vi "LVJSON Set.vi"(8 "error in (no error)":errorcluster, 10 "Root Element to Merge":T1, 11 "Root Element in":T1) -> (0 "error out":errorcluster, 2 "Exists?":bool, 3 "Root Element out":T1)   [LabVIEW 2019, in "labview_json.lvlib"]
uses:
  labview_json.lvlib
  Element.ctl
  Element Type.ctl
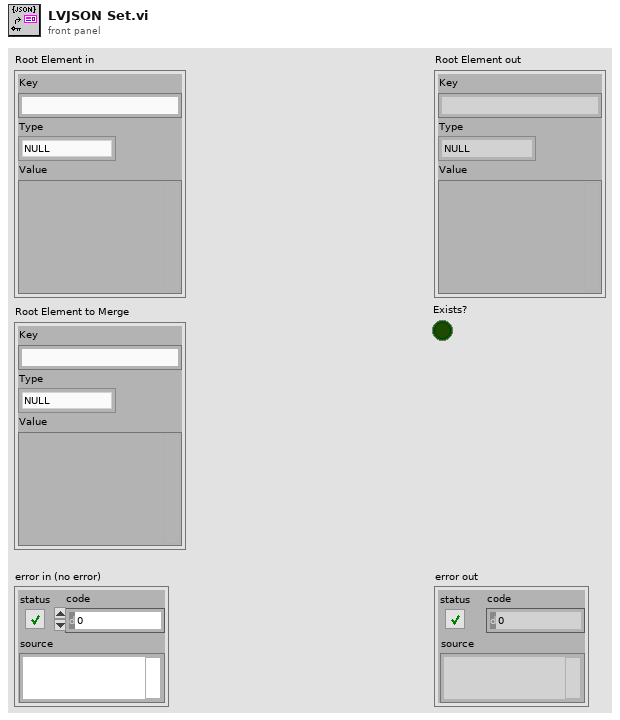
[diagram p1: front panel]
types:
  T1 = typedef "labview_json.lvlib/Element.ctl" = cluster{"Key":string, "Type":T2, "Value":variant}
  T2 = typedef "labview_json.lvlib/Element Type.ctl" = enum8{"NULL", "BOOL", "INT", "UINT", "FLOAT", "STRING", "ARRAY", "OBJECT", "SKIP"}
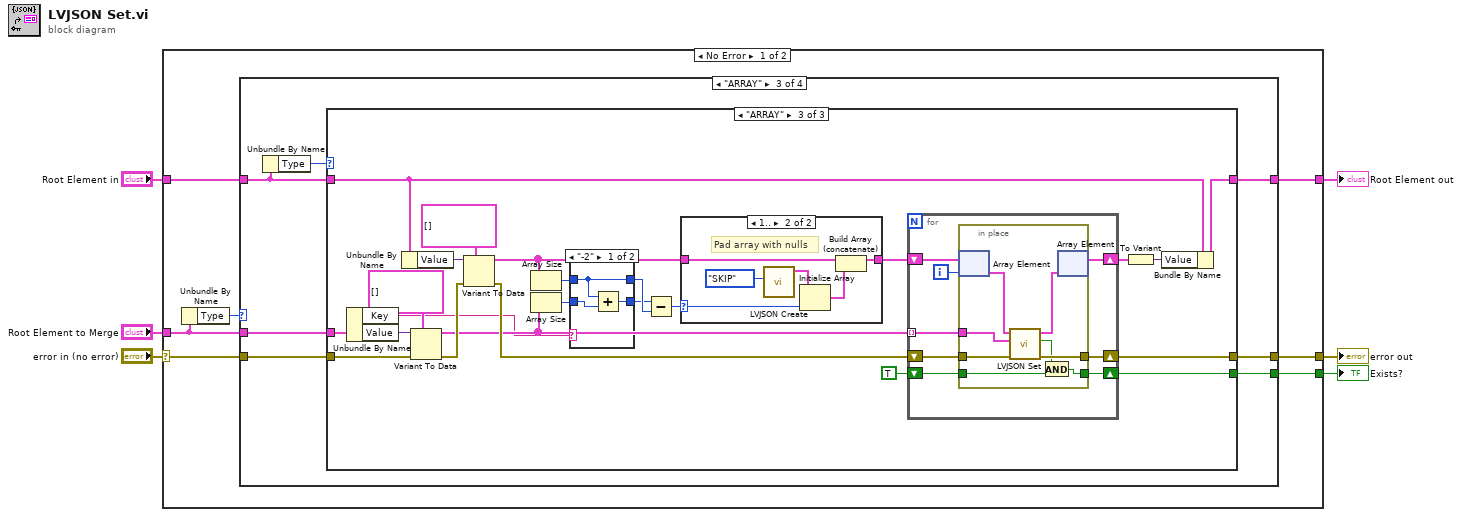
[diagram p0: block diagram]
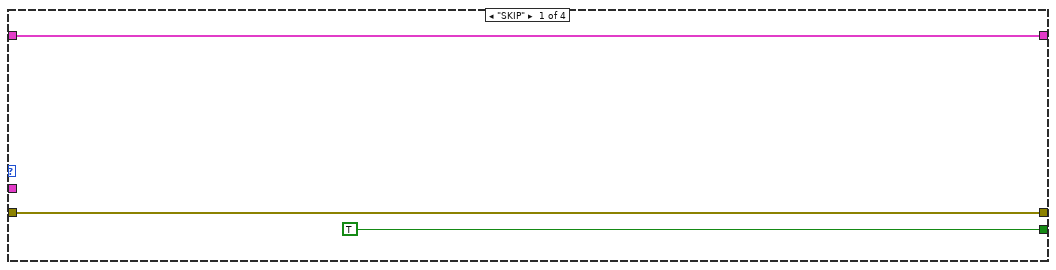
[diagram p2: hidden frame]
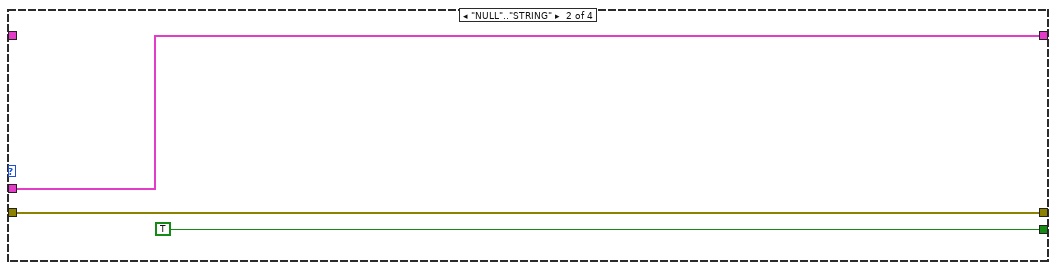
[diagram p3: hidden frame]
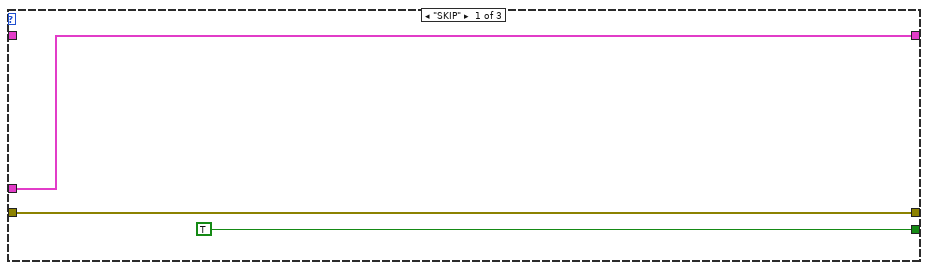
[diagram p4: hidden frame]
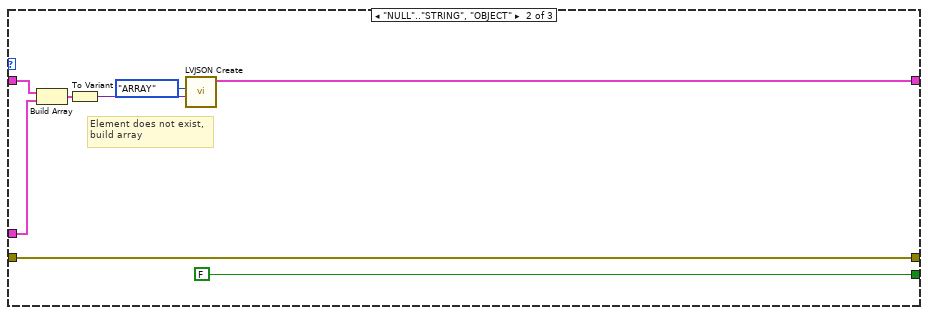
[diagram p5: hidden frame]
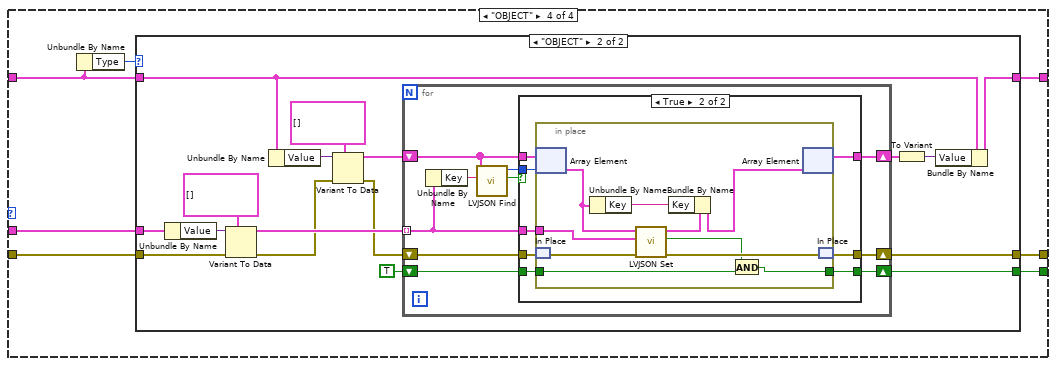
[diagram p8: hidden frame]
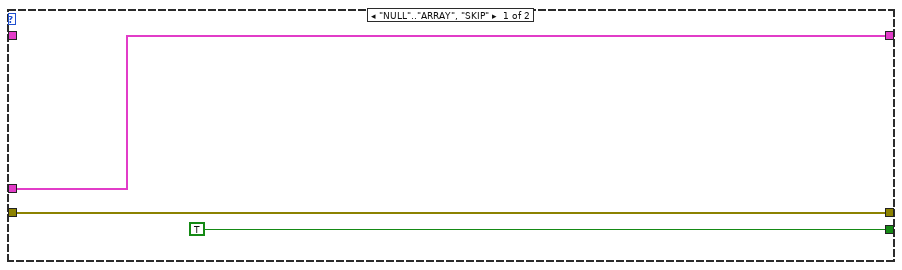
[diagram p9: hidden frame]
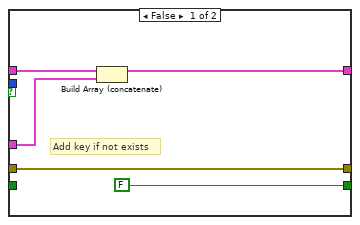
[diagram p10: hidden frame]
diagram:
  n1 = case shown="No Error" "error in (no error)" {
    selector: "error in (no error)" -> [w8 w151]
    tunnel: [w11 w151] -> w6
    tunnel: "Root Element in" -> [w13 w150]
    tunnel: "Root Element to Merge" -> [w7 _]
    tunnel: [w12 w150] -> w2
    tunnel: [w10 _] -> w1
    frame No Error {
      n2 = Unbundle By Name(w7) -> ("Type"=w9:T2)
      n3 = case shown="\"ARRAY\"" w9 {
        tunnel: w13 -> [w16 _ w22 w90]
        tunnel: [w16 w17 w25 w95] -> w12
        tunnel: w7 -> [_ w17 w20 w93]
        tunnel: w8 -> [w15 w19 w21 w91]
        tunnel: [w15 w19 w26 w96] -> w11
        tunnel: [TRUE ("Exists?") TRUE ("Exists?") w24 w94] -> w10
        frame "SKIP" {
        }
        frame "NULL".."STRING" {
        }
        frame "ARRAY" {
          n4 = Unbundle By Name(w22) -> ("Type"=w23:T2)
          n5 = case shown="\"ARRAY\"" w23 {
            tunnel: w22 -> [_ w37 w54]
            tunnel: w21 -> [w28 w36 w47]
            tunnel: [w28 w36 w61] -> w26
            tunnel: [w29 w35 w60] -> w25
            tunnel: [TRUE ("Exists?") FALSE ("Exists?") w59] -> w24
            tunnel: w20 -> [w29 w30 w46]
            frame "SKIP" {
            }
            frame "NULL".."STRING", "OBJECT" {
              # "Element does not exist,\nbuild array"
              n6 = Build Array(w37, w30) -> (w33:T1[])
              n7 = To Variant(anything=w33) -> (Variant=w32:variant)
              n8 = call "LVJSON Create.vi"("Variant (Void=Default Type)"=w32, "Type"=Element_Type."ARRAY") -> ("Element out"=w35:T1)  [unwired: 9 in]
            }
            frame "ARRAY" {
              n9 = Unbundle By Name(w46) -> ("Key"=w42:string, "Value"=w51:variant)
              n10 = Unbundle By Name(w54) -> ("Value"=w58:variant)
              n11 = Variant To Data(error in=w47, type=T1[] [], Variant=w51) -> (data=w48:T1[], error out=w49:errorcluster)
              n12 = Variant To Data(error in=w49, type=T1[] [], Variant=w58) -> (data=w53:T1[], error out=w52:errorcluster)
              n13 = Array Size(array=w53) -> (size(s)=w40:i32)
              n14 = Array Size(array=w48) -> (size(s)=w38:i32)
              n15 = case shown="\"-2\"" w42 {
                tunnel: [w63 w66] -> w41
                tunnel: w40 -> [w63 w66]
                tunnel: [w64 w65] -> w39
                tunnel: w38 -> [w62 w65]
                frame "-2" {
                  n16 = Add(x=w63, y=w62) -> (x+y=w64:i32)
                }
                frame Default {
                }
              }
              n17 = Subtract(x=w39, y=w41) -> (x-y=w44:i32)
              n18 = case shown="1.." w44 {
                selector: w44 -> [_ w68]
                tunnel: w53 -> [w67 w70]
                tunnel: [w67 w69] -> w45
                frame ..0 {
                }
                frame 1.. {
                  # "Pad array with nulls"
                  n19 = call "LVJSON Create.vi"("Type"=Element_Type."SKIP") -> ("Element out"=w72:T1)  [unwired: 10 in]
                  n20 = Initialize Array(w72, w68) -> (w71:T1[])
                  n21 = Build Array (concatenate)(w70, w71) -> (w69:T1[])
                }
              }
              n22 = for {
                tunnel: w48 -> [w74] mode=indexing
                shift-right: [w78] -> w61
                shift-left: w52 -> [w79]
                shift-right: [w77] -> w55
                shift-left: w45 -> [w81]
                shift-right: [w80] -> w59
                shift-left: TRUE ("Exists?") -> [w75]
                i -> [w76]
                n23 = in-place {
                  in-place-border: w79 -> [w89]
                  in-place-border: [w88] -> w78
                  in-place-border: [w83] -> w80
                  in-place-border: w74 -> [w82]
                  in-place-border: w75 -> [w84]
                  n24 = in-place-array #1(w81, w76) -> (w86:T1)
                  n25 = call "LVJSON Set.vi"("error in (no error)"=w89, "Root Element to Merge"=w82, "Root Element in"=w86) -> ("error out"=w88:errorcluster, "Exists?"=w85:bool, "Root Element out"=w87:T1)  [unwired: 6 in]
                  n26 = And(x=w85, y=w84) -> (x .and. y?=w83:bool)
                  n27 = in-place-array #1(w87) -> (w77:T1[])  [unwired: 1 out]
                }
              }
              n28 = To Variant(anything=w55) -> (Variant=w56:variant)
              n29 = Bundle By Name(cluster=w54, "Value"=w56) -> (w60:T1)
            }
          }
        }
        frame "OBJECT" {
          n30 = Unbundle By Name(w90) -> ("Type"=w92:T2)
          n31 = case shown="\"OBJECT\"" w92 {
            tunnel: w91 -> [w99 w102]
            tunnel: w90 -> [_ w103]
            tunnel: [w99 w116] -> w96
            tunnel: [w97 w115] -> w95
            tunnel: [TRUE ("Exists?") w114] -> w94
            tunnel: w93 -> [w97 w113]
            frame "NULL".."ARRAY", "SKIP" {
            }
            frame "OBJECT" {
              n32 = Unbundle By Name(w113) -> ("Value"=w112:variant)
              n33 = Variant To Data(error in=w102, type=T1[] [], Variant=w112) -> (data=w111:T1[], error out=w101:errorcluster)
              n34 = Unbundle By Name(w103) -> ("Value"=w106:variant)
              n35 = Variant To Data(error in=w101, type=T1[] [], Variant=w106) -> (data=w104:T1[], error out=w100:errorcluster)
              n36 = for {
                tunnel: w111 -> [w123] mode=indexing
                shift-right: [w120] -> w116
                shift-left: w100 -> [w121]
                shift-right: [w124] -> w109
                shift-left: w104 -> [w125]
                shift-right: [w122] -> w114
                shift-left: TRUE ("Exists?") -> [w118]
                n37 = Unbundle By Name(w123) -> ("Key"=w117:string)
                n38 = call "LVJSON Find.vi"("Key"=w117, "Elements in"=w125) -> ("Found?"=w126:bool, "Index"=w119:i32)  [unwired: 8 in]
                n39 = case shown="True" w126 {
                  tunnel: w125 -> [w131 w139]
                  tunnel: w119 -> [_ w138]
                  tunnel: w123 -> [w128 w134]
                  tunnel: [w130 w137] -> w124
                  tunnel: [FALSE w133] -> w122
                  tunnel: w121 -> [w129 w136]
                  tunnel: [w129 w135] -> w120
                  tunnel: w118 -> [_ w132]
                  frame False {
                    # "Add key if not exists"
                    n40 = Build Array (concatenate)(w131, w128) -> (w130:T1[])
                  }
                  frame True {
                    n41 = in-place {
                      in-place-border: w134 -> [w140]
                      in-place-border: [w144] -> w133
                      in-place-border: w132 -> [w146]
                      n42 = in-place-array #2(w139, w138) -> (w142:T1)
                      n43 = in-place-match #3(w136) -> (w149:errorcluster)
                      n44 = Unbundle By Name(w142) -> ("Key"=w141:string)
                      n45 = call "LVJSON Set.vi"("error in (no error)"=w149, "Root Element to Merge"=w140, "Root Element in"=w142) -> ("error out"=w147:errorcluster, "Exists?"=w145:bool, "Root Element out"=w148:T1)  [unwired: 6 in]
                      n46 = Bundle By Name(cluster=w148, "Key"=w141) -> (w143:T1)
                      n47 = And(x=w145, y=w146) -> (x .and. y?=w144:bool)
                      n48 = in-place-array #2(w143) -> (w137:T1[])  [unwired: 1 out]
                      n49 = in-place-match #3(w147) -> (w135:errorcluster)
                    }
                  }
                }
              }
              n50 = To Variant(anything=w109) -> (Variant=w110:variant)
              n51 = Bundle By Name(cluster=w103, "Value"=w110) -> (w115:T1)
            }
          }
        }
      }
    }
    frame Error {
    }
  }
  "error out" <- w6
  "Exists?" <- w1
  "Root Element out" <- w2
